vi "Update Filing Info.vi"(6 "Location":string, 8 "error in (no error)":errorcluster, 11 "Worker in":refnum<class "Worker Actor.lvclass">) -> (0 "error out":errorcluster, 3 "Worker out":refnum<class "Worker Actor.lvclass">)   [LabVIEW 2024, in "Worker Actor.lvclass"]
uses:
  Worker Actor.lvclass
  Worker Actor.lvclass/Worker Actor.ctl
  Write Project folder .vi
  Write File middle.vi
  NHMFL_Core/Libraries/File/Metadata/Metadata.lvclass
panel:
  out "PI":string
  out "Experiment":string
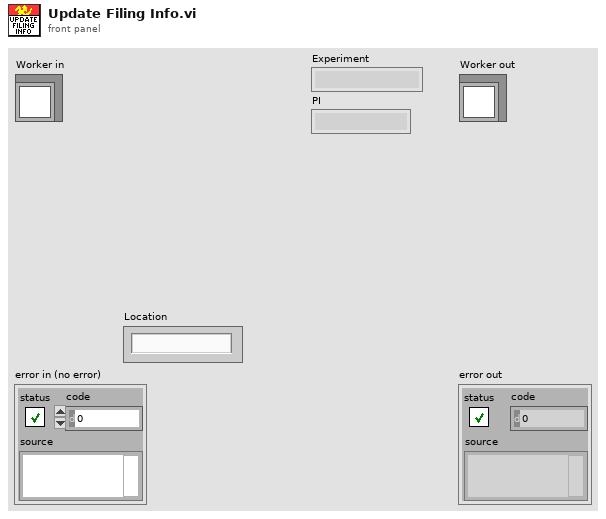
[diagram p1: front panel]
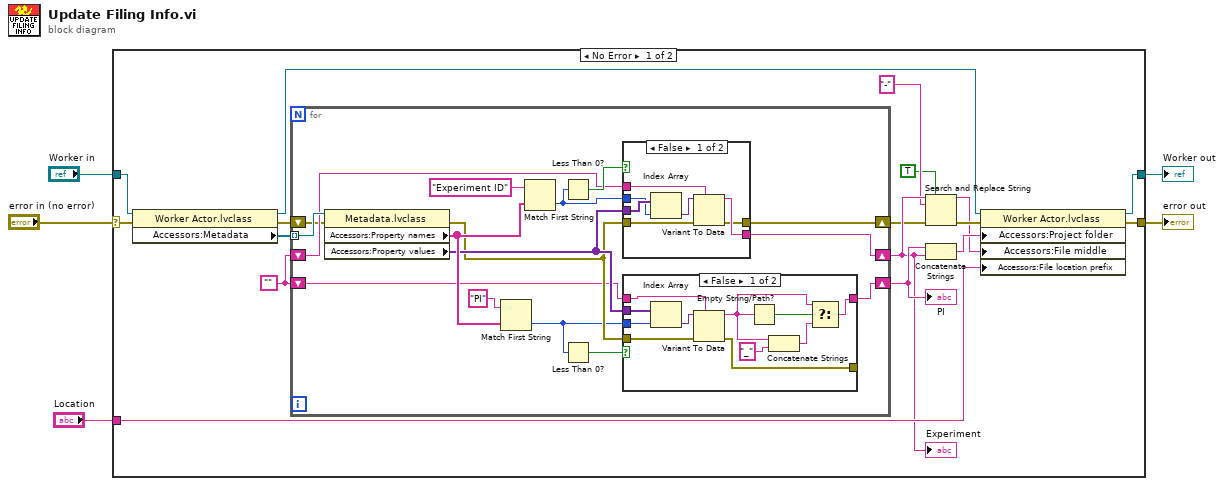
[diagram p0: block diagram]
diagram:
  n1 = case shown="No Error" "error in (no error)" {
    selector: "error in (no error)" -> [w22 w62]
    tunnel: [w13 w62] -> w4
    tunnel: [w16 w61] -> w2
    tunnel: "Worker in" -> [w20 w61]
    tunnel: "Location" -> [w12 _]
    frame No Error {
      w17 = ""
      n2 = property class="Worker Actor.lvclass"(reference=w20, error in=w22) -> (reference out=w19:refnum<class "Worker Actor.lvclass">, error out=w21:errorcluster, "Accessors:Metadata"=w18:refnum<class "Metadata.lvclass">[])
      n3 = for {
        tunnel: w18 -> [w38] mode=indexing
        shift-right: [w23] -> w15
        shift-left: w17 -> [w24]
        shift-right: [w33] -> w11
        shift-left: w17 -> [w34]
        shift-right: [w32] -> w9
        shift-left: w21 -> [w31]
        n4 = property class="Metadata.lvclass"(reference=w38, error in=w31) -> (error out=w26:errorcluster, "Accessors:Property names"=w29:string[], "Accessors:Property values"=w27:variant[])  [unwired: 1 out]
        n5 = Match First String(2:w29, 3:"PI" ("string")) -> (0:w25:i32)  [unwired: 1 out]
        n6 = Match First String(2:w29, 3:"Experiment ID" ("string")) -> (0:w35:i32)  [unwired: 1 out]
        n7 = Less Than 0?(x=w35) -> (x < 0?=w36:bool)
        n8 = Less Than 0?(x=w25) -> (x < 0?=w28:bool)
        n9 = case shown="False" w36 {
          tunnel: w27 -> [w58 _]
          tunnel: w35 -> [w56 _]
          tunnel: w34 -> [w55 w60]
          tunnel: [w54 w60] -> w33
          tunnel: [w52 w59] -> w32
          tunnel: w26 -> [w53 w59]
          frame False {
            n10 = Index Array(array=w58, index=w56) -> (element=w57:variant)
            n11 = Variant To Data(error in=w53, type=w55, Variant=w57) -> (data=w54:string, error out=w52:errorcluster)
          }
          frame True {
          }
        }
        n12 = case shown="False" w28 {
          tunnel: w27 -> [w49 _]
          tunnel: w25 -> [w47 _]
          tunnel: w24 -> [w46 w51]
          tunnel: [w39 w51] -> w23
          tunnel: [w44 w50] -> _
          tunnel: w26 -> [w45 w50]
          frame False {
            n13 = Index Array(array=w49, index=w47) -> (element=w48:variant)
            n14 = Variant To Data(error in=w45, type=w46, Variant=w48) -> (data=w41:string, error out=w44:errorcluster)
            n15 = Empty String/Path?(string/path=w41) -> (empty?=w42:bool)
            n16 = Concatenate Strings(w41, "_" ("string")) -> (w40:string)
            n17 = Select(t=w41, s=w42, f=w40) -> (s? t:f=w39:string)
          }
          frame True {
          }
        }
      }
      "Experiment" <- w11
      "PI" <- w15
      n18 = Search and Replace String(replace all?=TRUE ("replace all? (F)"), input string=w11, search string="-", error in=w9) -> (result string=w7:string, error out=w8:errorcluster)  [unwired: 4 in, 2 out]
      n19 = Concatenate Strings(w15, w11) -> (w14:string)
      n20 = property class="Worker Actor.lvclass"(reference=w19, error in=w8, "Accessors:Project folder "=w14, "Accessors:File middle"=w7, "Accessors:File location prefix"=w12) -> (reference out=w16:refnum<class "Worker Actor.lvclass">, error out=w13:errorcluster)
    }
    frame Error {
    }
  }
  "error out" <- w4
  "Worker out" <- w2
